vi "main_v1.1.vi"() -> ()   [LabVIEW 2012]
uses:
  SensorSettingCtl.ctl
  SensorTypes.ctl
  states.ctl
  globalVariables.vi
  <vilib>/Analysis/baseanly.llb/Mean (DBL).vi
  <vilib>/Analysis/NI_AALBase.lvlib
panel:
  out "times":dbl[](array[numeric])
  out "diff":dbl
  in  "max. meas. time / ms":dbl=3000.0
  out "means":dbl[](array[numeric])
  out "measuring":bool
  out "i_e":i32
  out "i_s":i32
  out "XY Graph raw":cluster{dbl[], dbl[]}[](graph)
  out "XY Graph":cluster{dbl[], dbl[]}[](graph)
  in  "size of buffer":i32=1000000
  in  "Path for measuring results":path=path "C:/Users/Induelec/Desktop/test_output"
  in  "Sensor types":T1[](array[typedef])=[enum."ITL 900 (Analogue)", enum."CAB 300-C SP3 (CAN)", enum."xyz TODO (PWM)", enum."xyz TODO (LIN)", enum."xyz TODO (Analogue)"]
  in  "Array 2":T2[](array[typedef])=[{"VISA resource name"="", "use sensor"=FALSE}, {"VISA resource name"="", "use sensor"=TRUE}, {"VISA resource name"="", "use sensor"=FALSE}, {"VISA resource name"="", "use sensor"=FALSE}, {"VISA resource name"="", "use sensor"=FALSE}]
  in  "cancel button":bool
  in  "start Button":bool
  out "Error Flag":bool
  # "Measurement of Current Sensors from LEM"
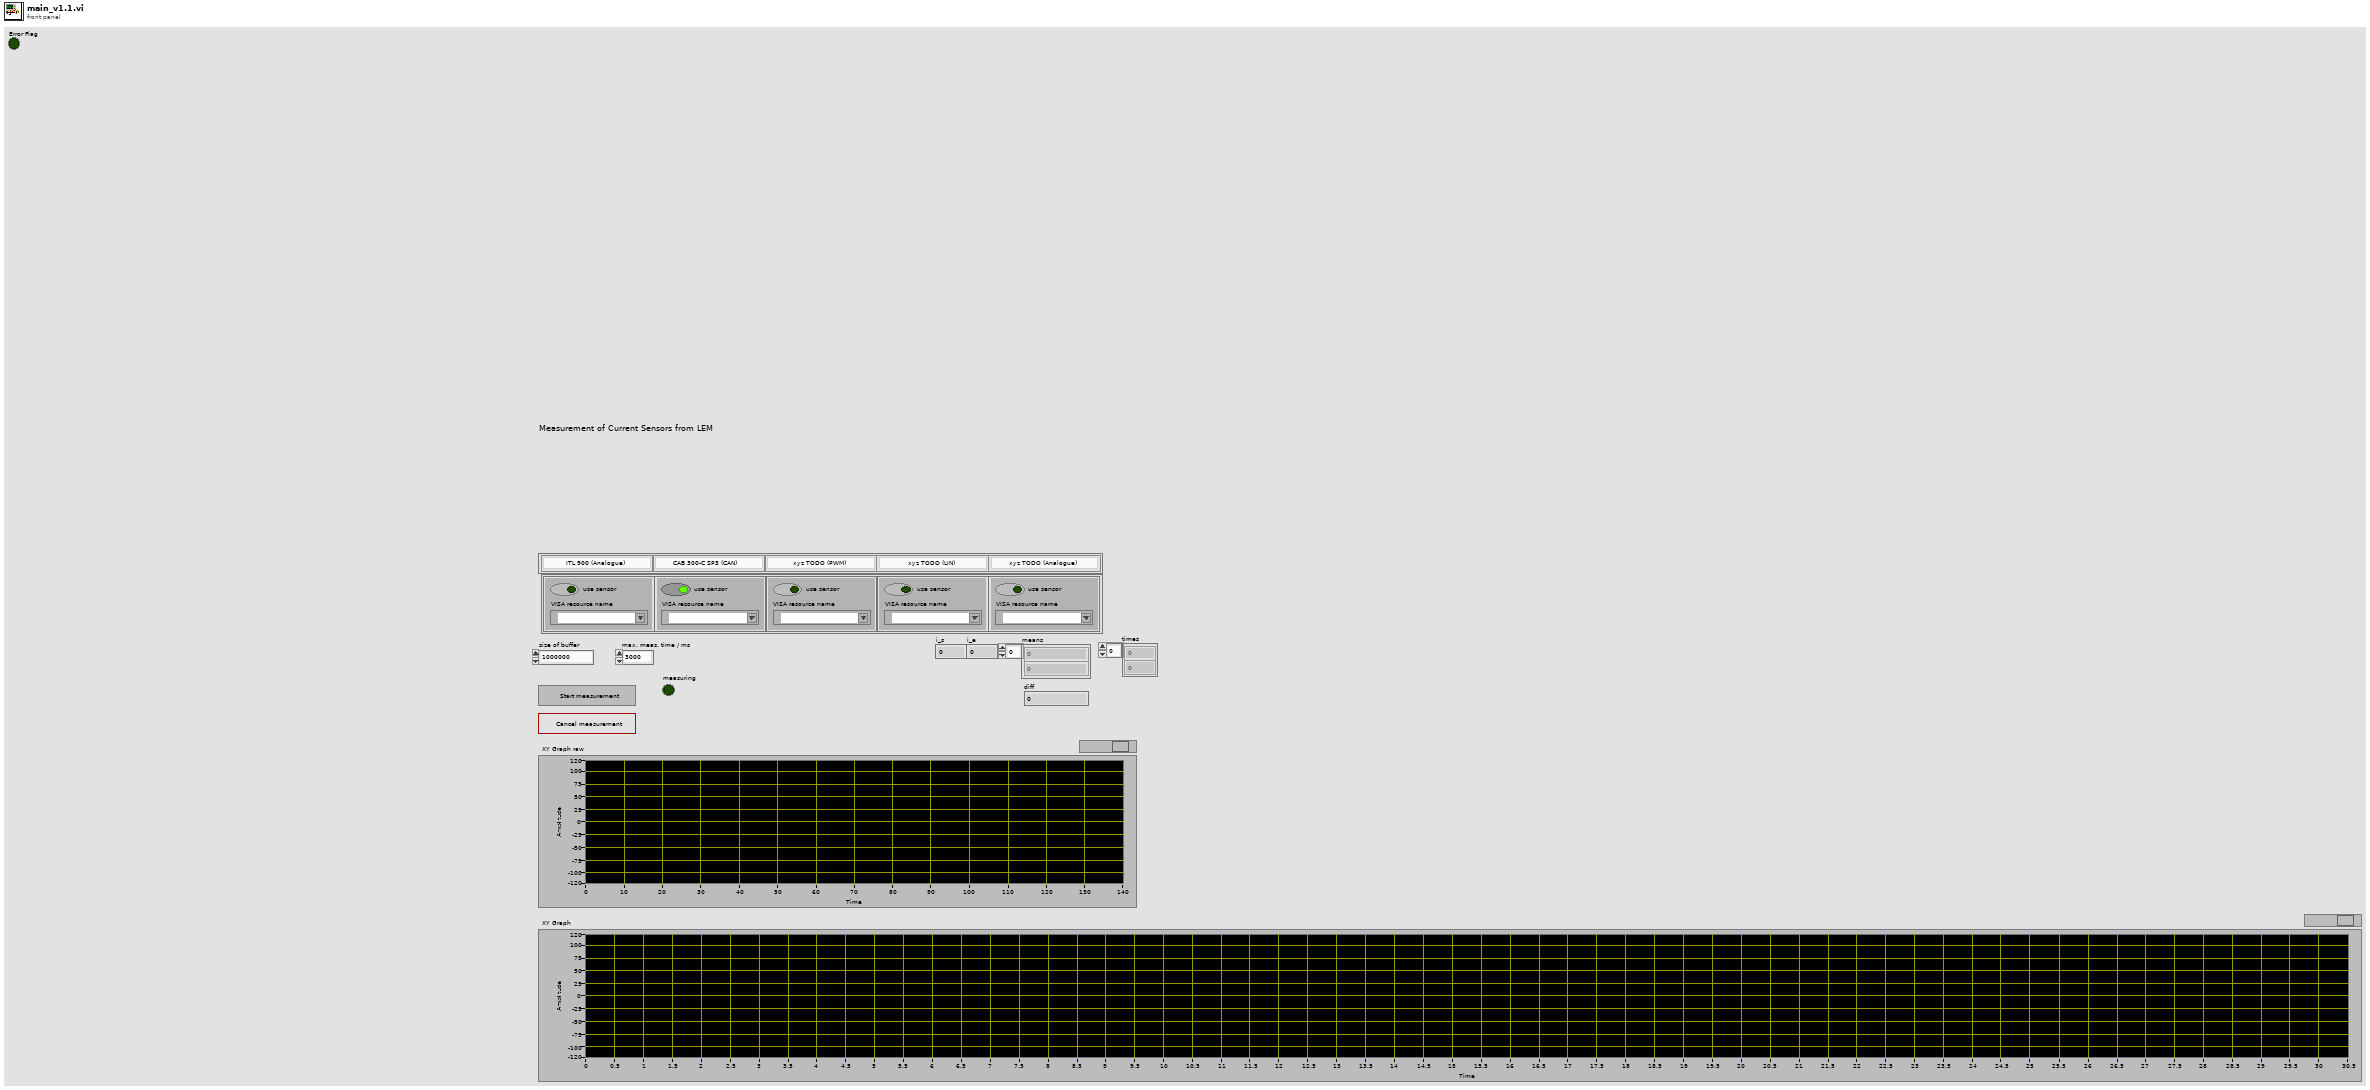
[diagram p1: front panel]
types:
  T1 = typedef "SensorTypes.ctl" = enum16{"ITL 900 (Analogue)", "CAB 300-C SP3 (CAN)", "xyz TODO (PWM)", "xyz TODO (LIN)", "xyz TODO (Analogue)"}
  T2 = typedef "SensorSettingCtl.ctl" = cluster{"VISA resource name":refnum<visa-resource-name>, "use sensor":bool}
  T3 = typedef "states.ctl" = enum16{"init", "wait for user confirm", "start sensors", "measure", "data analysis", "terminate"}
  T4 = typedef "TimeValue.ctl" = cluster{"Time of measurement":timestamp, "Current value":dbl}
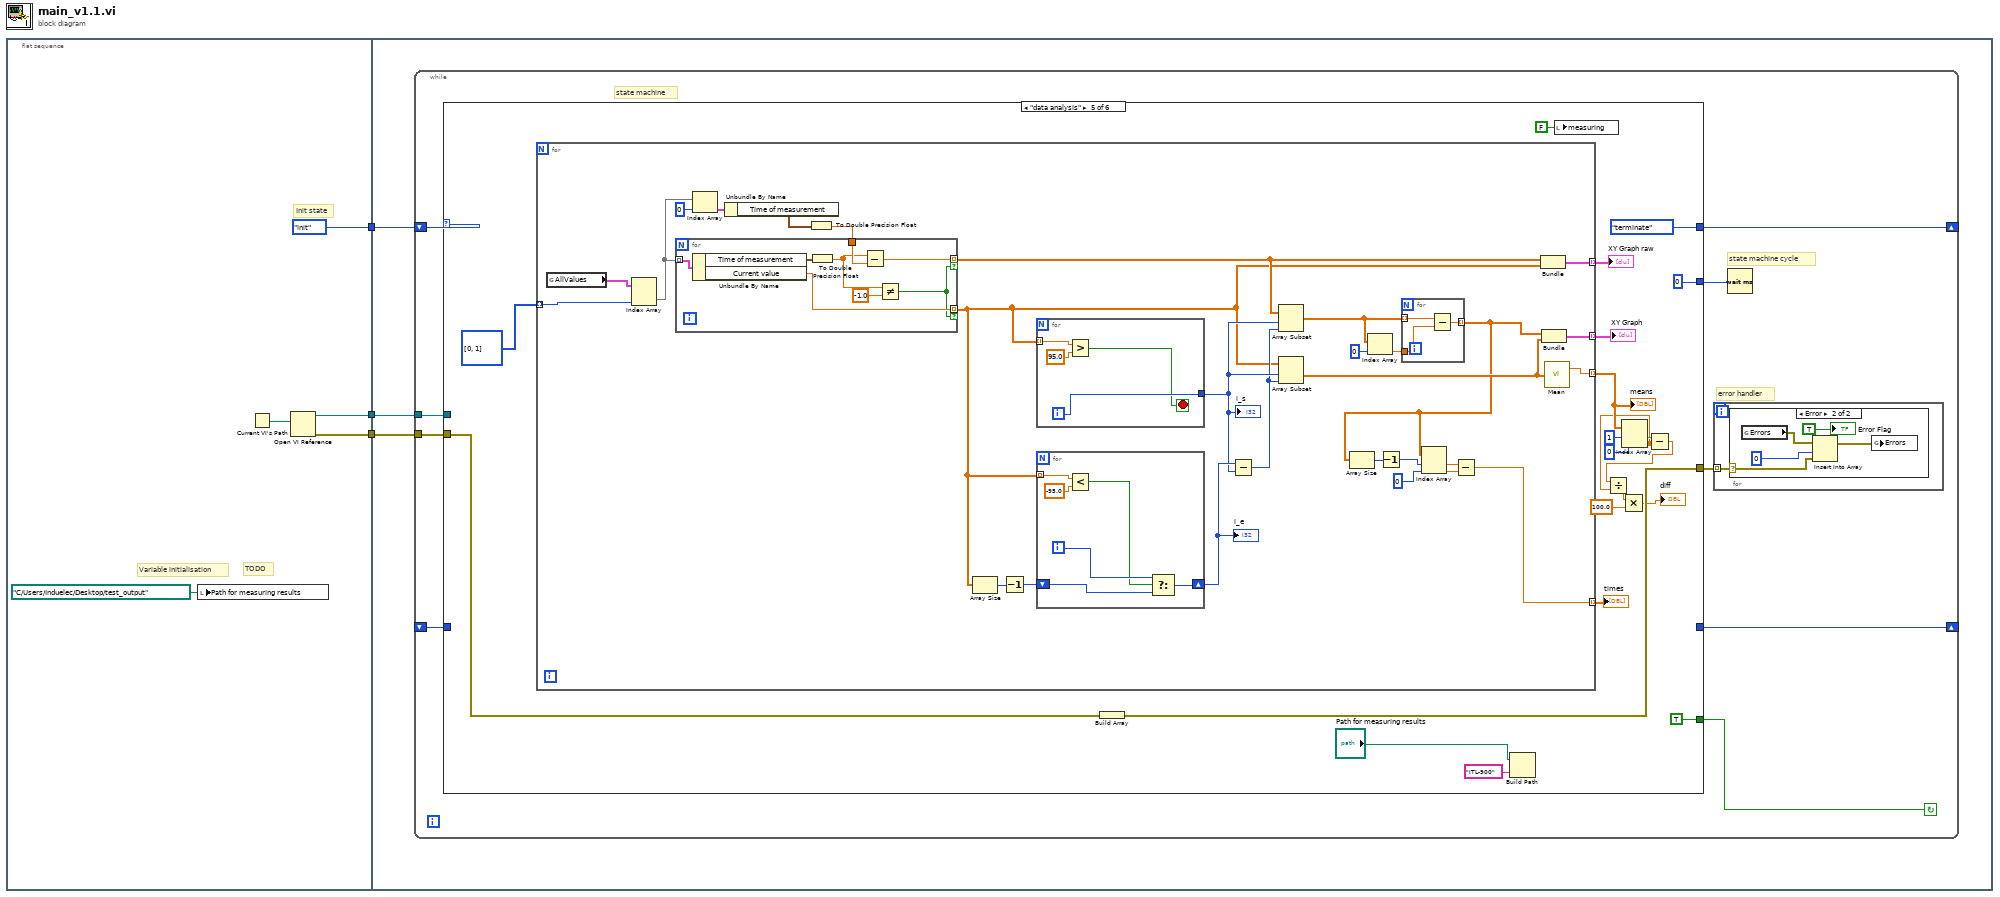
[diagram p0: block diagram]
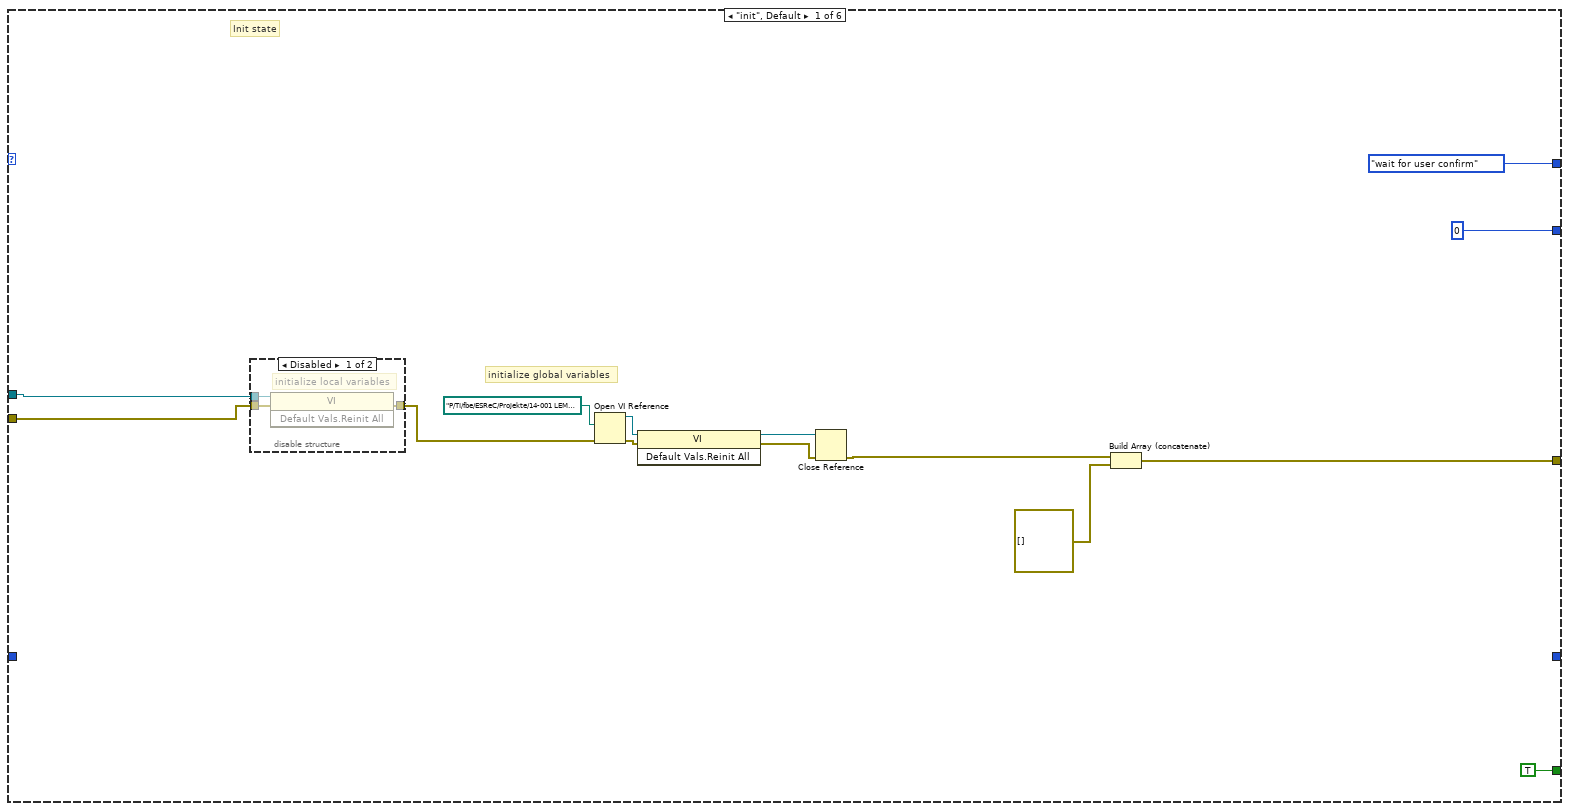
[diagram p3: hidden frame]
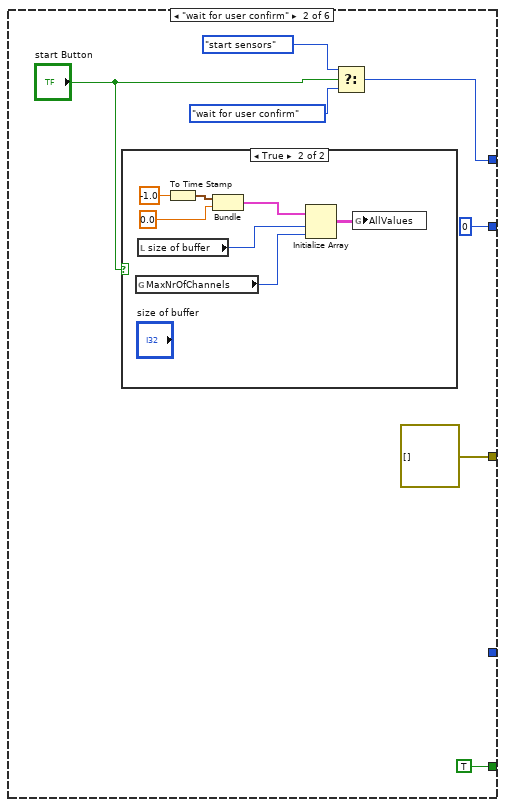
[diagram p5: hidden frame]
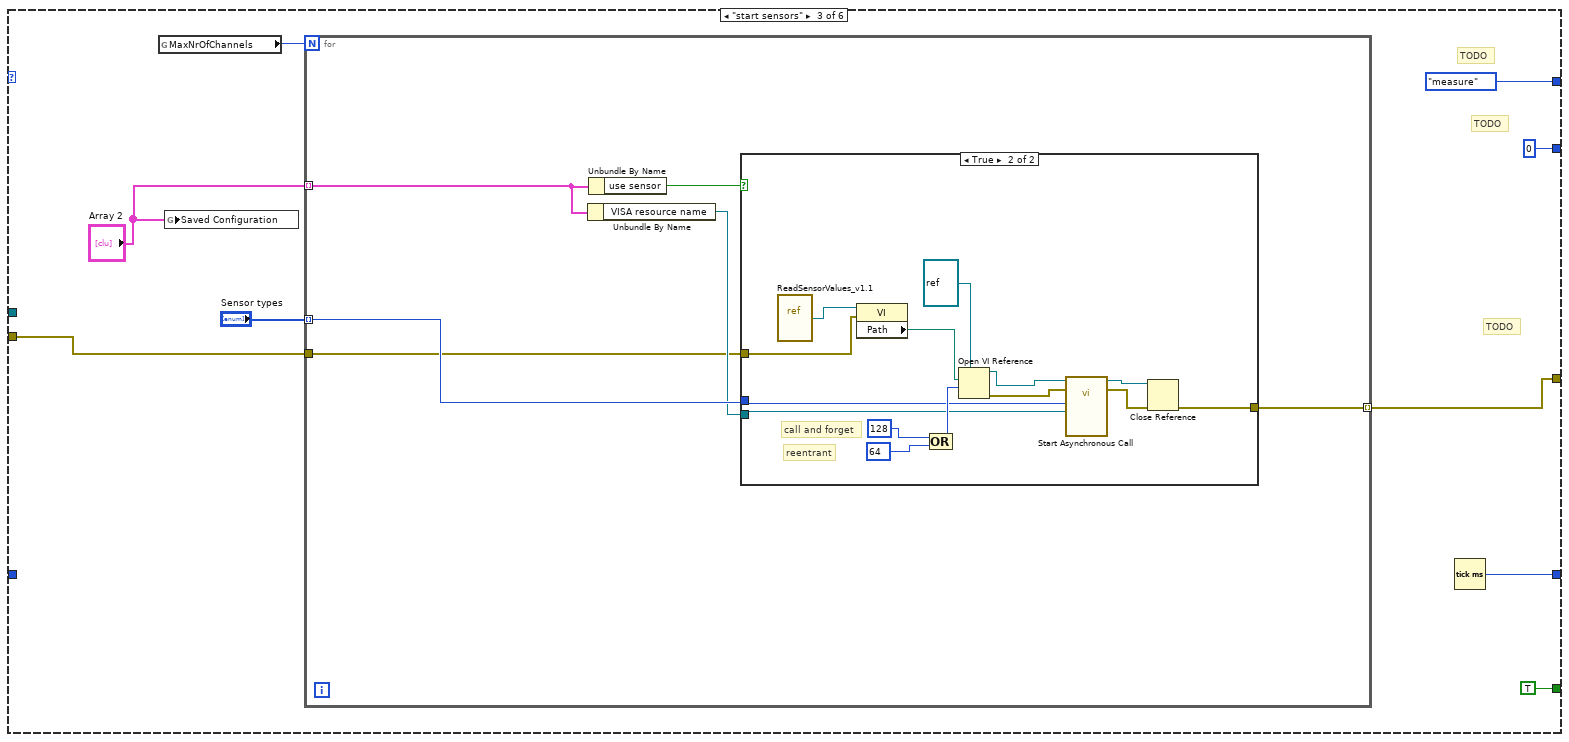
[diagram p7: hidden frame]
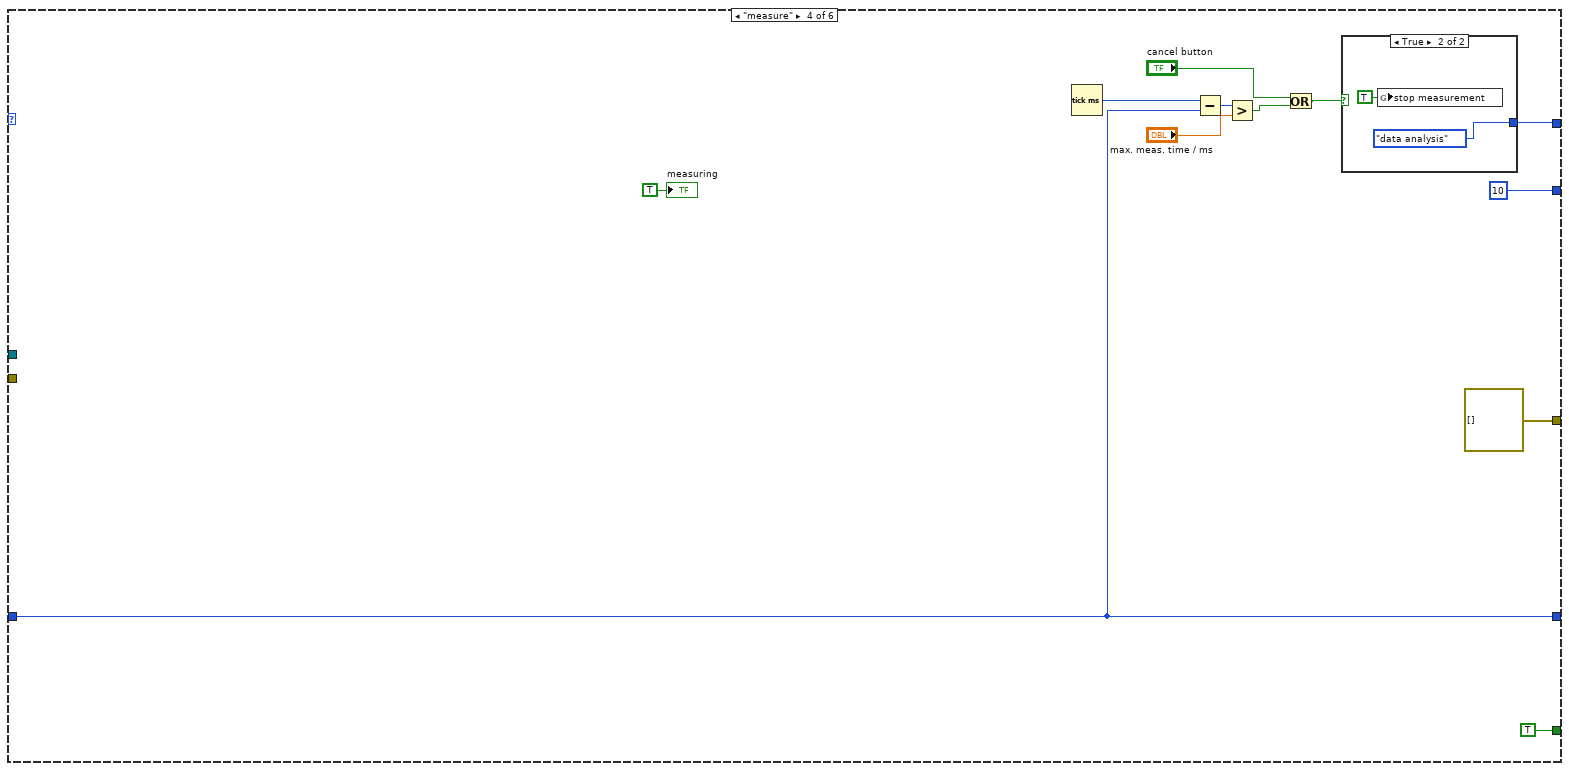
[diagram p9: hidden frame]
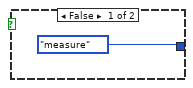
[diagram p10: hidden frame]
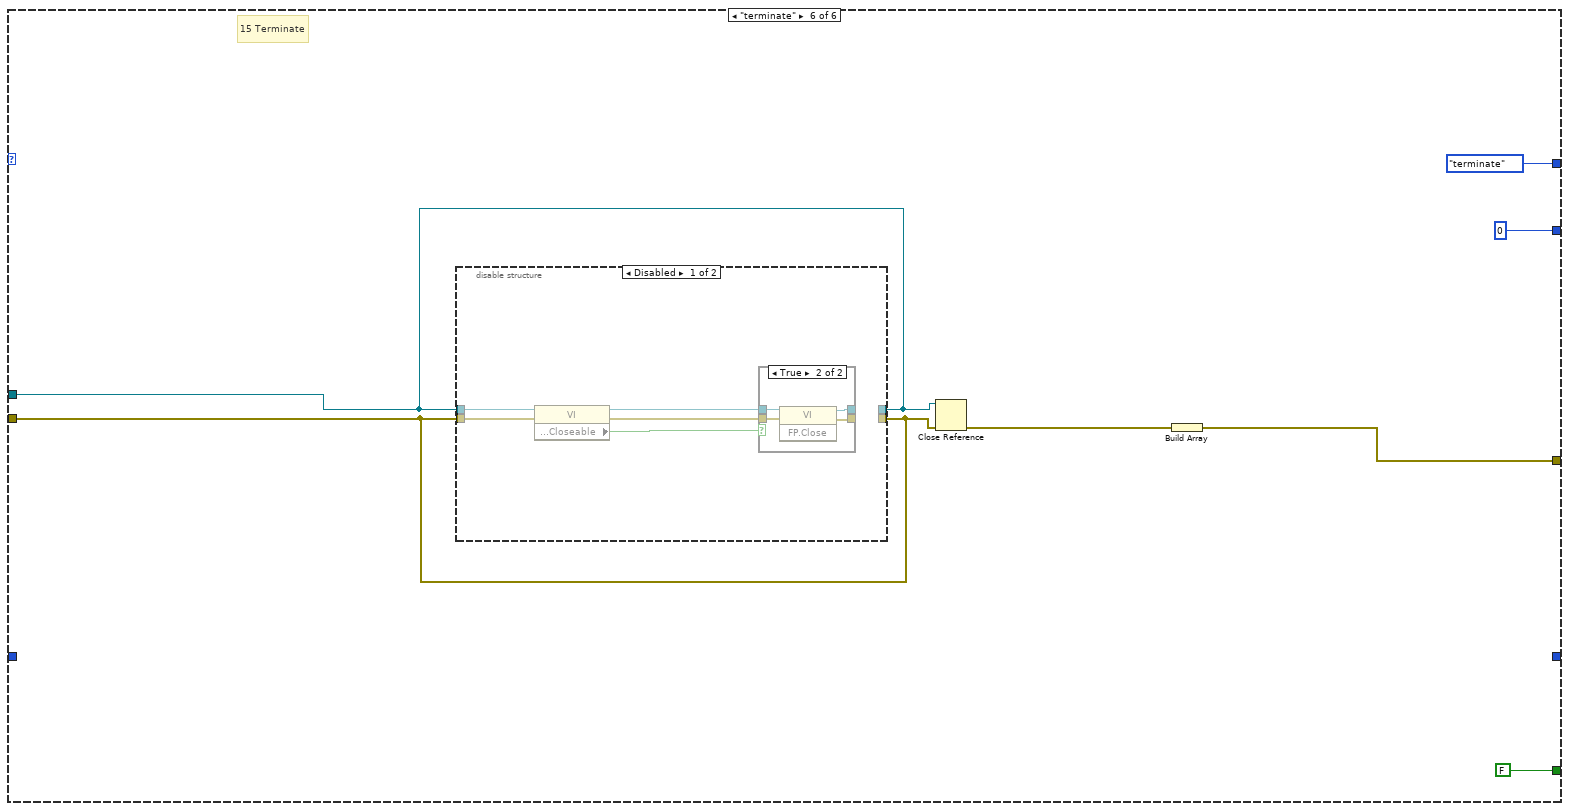
[diagram p11: hidden frame]
diagram:
  n1 = flat-sequence {
    tunnel: [states."init" ("States IEEE-488")] -> w3
    tunnel: [w8] -> w2
    tunnel: [w7] -> w1
    tunnel: w3 -> [w9]
    tunnel: w2 -> [w11]
    tunnel: w1 -> [w10]
    frame #0 {
      # "TODO"
      # "Variable initialisation"
      # "Init state"
      n2 = local write "Path for measuring results"(path "C:/Users/Induelec/Desktop/test_output" ("Path for measuring results")) -> ()
      n3 = Current VI's Path() -> (path=w6:path)
      n4 = Open VI Reference(vi path=w6) -> (vi reference=w8:refnum<vi>, error out=w7:errorcluster)  [unwired: 2 in, 3 out]
    }
    frame #1 {
      n5 = while {
        tunnel: w11 -> [w19]
        tunnel: w10 -> [w18]
        shift-right: [w15] -> _
        shift-left: w9 -> [w16]
        shift-right: [w13] -> _
        shift-left: _ -> [w12]
        stop <- w14 continue-if-true
        # "state machine"
        # "error handler"
        # "state machine cycle"
        n6 = case shown="\"data analysis\"" w16 {
          tunnel: [u32 0 ("milliseconds to wait") u32 0 ("milliseconds to wait") u32 0 ("milliseconds to wait") u32 10 ("milliseconds to wait") u32 0 ("milliseconds to wait") u32 0 ("milliseconds to wait")] -> w20
          tunnel: w19 -> [w37 _ _ _ _ w174]
          tunnel: w18 -> [w38 _ w59 _ w118 w173]
          tunnel: [w39 errorcluster[] [] w64 errorcluster[] [] w119 w178] -> w17
          tunnel: [states."wait for user confirm" ("States IEEE-488") w48 states."measure" ("States IEEE-488") w98 states."terminate" ("f") states."terminate" ("f")] -> w15
          tunnel: [TRUE TRUE TRUE TRUE TRUE FALSE] -> w14
          tunnel: [_ _ w58 w89 _ _] -> w13
          tunnel: w12 -> [_ _ _ w89 _ _]
          frame "init", Default {
            # "initialize global variables"
            # "Init state"
            n7 = disable-structure shown="Disabled" {
              disable-tunnel: w38 -> [w43 _]
              disable-tunnel: w37 -> [w42 _]
              disable-tunnel: [w41 _] -> w31
              frame Disabled {
                # "initialize local variables"
                n8 = invoke class="VI" method="Default Vals.Reinit All"(reference=w42, error in=w43) -> (error out=w41:errorcluster)  [unwired: 1 in, 2 out]
              }
              frame Enabled {
              }
            }
            n9 = Open VI Reference(vi path=path "P:/TI/fbe/ESReC/Projekte/14-001 LEM Current Sensor Measurements/Software/LabVIEW/Current sensor tests/globalVariables.vi", error in (no error)=w31) -> (vi reference=w32:refnum<vi>, error out=w30:errorcluster)  [unwired: 4 in]
            n10 = invoke class="VI" method="Default Vals.Reinit All"(reference=w32, error in=w30) -> (reference out=w29:refnum<vi>, error out=w28:errorcluster)  [unwired: 1 in, 1 out]
            n11 = Close Reference(reference=w29, error in (no error)=w28) -> (error out=w27:errorcluster)
            n12 = Build Array (concatenate)(w27, errorcluster[] [] ("array")) -> (w39:errorcluster[])
          }
          frame "wait for user confirm" {
            n13 = case shown="True" "start Button" {
              frame False {
              }
              frame True {
                n14 = global read "globalVariables.vi" "MaxNrOfChannels"() -> (w57:i32)
                n15 = local read "size of buffer"() -> (w55:i32)
                n16 = To Time Stamp(1:-1.0 ("number")) -> (0:w53:timestamp)
                n17 = Bundle(w53, 0.0) -> (w51:cluster{timestamp, dbl})  [unwired: 1 in]
                n18 = Initialize Array(w51, w55, w57) -> (w56:cluster{timestamp, dbl}[][])
                n19 = global write "globalVariables.vi" "AllValues"(w56) -> ()
              }
            }
            n20 = Select(t=states."start sensors" ("States IEEE-488"), s="start Button", f=states."wait for user confirm" ("States IEEE-488")) -> (s? t:f=w48:T3)
          }
          frame "start sensors" {
            # "TODO"
            # "TODO"
            # "TODO"
            n21 = global read "globalVariables.vi" "MaxNrOfChannels"() -> (w61:i32)
            n22 = global write "globalVariables.vi" "Saved Configuration"("Array 2") -> ()
            n23 = for {
              N: w61 -> [_]
              tunnel: "Array 2" -> [w71] mode=indexing
              tunnel: [w70] -> w64 mode=indexing
              tunnel: "Sensor types" -> [w69] mode=indexing
              tunnel: w59 -> [w67]
              n24 = Unbundle By Name(w71) -> ("VISA resource name"=w68:refnum<visa-resource-name>)
              n25 = Unbundle By Name(w71) -> ("use sensor"=w72:bool)
              n26 = case shown="True" w72 {
                tunnel: [w73 w85] -> w70
                tunnel: w69 -> [_ w76]
                tunnel: w68 -> [_ w75]
                tunnel: w67 -> [w73 w77]
                frame False {
                }
                frame True {
                  # "reentrant"
                  # "call and forget"
                  n27 = vi-ref "ReadSensorValues_v1.1.vi"() -> (w78:refnum<vi>)
                  n28 = property class="VI"(reference=w78, error in=w77) -> ("Path"=w87:path)  [unwired: 2 out]
                  n29 = Compound Arithmetic op=OR(128 ("options"), 64 ("value")) -> (w84:i32)
                  n30 = Open VI Reference(type specifier VI Refnum (for type only)=refnum<vi> refnum, vi path=w87, options=w84) -> (vi reference=w82:refnum<vi>, error out=w81:errorcluster)  [unwired: 3 in]
                  n31 = call-by-ref "Start Asynchronous Call"(reference=w82, error in=w81, "VISA resource name"=w75, "Sensor type"=w76) -> (reference out=w80:refnum<vi>, error out=w79:errorcluster)  [unwired: 10 in]
                  n32 = Close Reference(reference=w80, error in (no error)=w79) -> (error out=w85:errorcluster)
                }
              }
            }
            n33 = Tick Count (ms)() -> (millisecond timer value=w58:u32)
          }
          frame "measure" {
            n34 = Tick Count (ms)() -> (millisecond timer value=w90:u32)
            n35 = Subtract(x=w90, y=w89) -> (x-y=w92:u32)
            n36 = Greater?(x=w92, y="max. meas. time / ms") -> (0:w93:bool)
            n37 = Or(x="cancel button", y=w93) -> (x .or. y?=w95:bool)
            n38 = case shown="True" w95 {
              tunnel: [states."measure" ("f") states."data analysis" ("States IEEE-488")] -> w98
              frame False {
              }
              frame True {
                n39 = global write "globalVariables.vi" "stop measurement"(TRUE ("stop measurement")) -> ()
              }
            }
            "measuring" <- TRUE ("measuring")
          }
          frame "data analysis" {
            n40 = for {
              tunnel: [w145] -> w114 mode=indexing
              tunnel: i32[] [0, 1] -> [w144] mode=indexing
              tunnel: [w138] -> w115 mode=indexing
              tunnel: [w133] -> w112 mode=indexing
              tunnel: [w126] -> w103 mode=indexing
              n41 = global read "globalVariables.vi" "AllValues"() -> (w151:T4[][])
              n42 = Index Array(array=w151, index (col)=w144) -> (element=w149:T4[])  [unwired: 1 in]
              n43 = Index Array(array=w149, index=0) -> (element=w148:T4)
              n44 = Unbundle By Name(w148) -> ("Time of measurement"=w147:timestamp)
              n45 = To Double Precision Float(number=w147) -> (double precision float=w146:dbl)
              n46 = for {
                tunnel: w149 -> [w172] mode=indexing
                tunnel: [w165] -> w137 mode=indexing if=w166
                tunnel: [w170] -> w132 mode=indexing if=w166
                tunnel: w146 -> [w169]
                n47 = Unbundle By Name(w172) -> ("Time of measurement"=w171:timestamp, "Current value"=w170:dbl)
                n48 = To Double Precision Float(number=w171) -> (double precision float=w167:dbl)
                n49 = Subtract(x=w167, y=w169) -> (x-y=w165:dbl)
                n50 = Not Equal?(x=w167, y=-1.0) -> (x != y?=w166:bool)
              }
              n51 = Array Size(array=w132) -> (size(s)=w143:i32)
              n52 = Decrement(x=w143) -> (x-1=w142:i32)
              n53 = for {
                tunnel: w132 -> [w164] mode=indexing
                tunnel: [w162] -> w140
                i -> [w162]
                stop <- w161 stop-if-true
                n54 = Greater?(x=w164, y=95.0) -> (0:w161:bool)
              }
              "i_s" <- w140
              n55 = for {
                tunnel: w132 -> [w160] mode=indexing
                shift-right: [w158] -> w141
                shift-left: w142 -> [w156]
                i -> [w157]
                n56 = Less?(x=w160, y=-95.0) -> (x < y?=w155:bool)
                n57 = Select(t=w157, s=w155, f=w156) -> (s? t:f=w158:i32)
              }
              "i_e" <- w141
              n58 = Subtract(x=w141, y=w140) -> (x-y=w139:i32)
              n59 = Array Subset(array=w137, index=w140, length=w139) -> (w136:dbl[])
              n60 = Array Subset(array=w132, index=w140, length=w139) -> (w131:dbl[])
              n61 = Index Array(array=w136, index=0) -> (element=w134:dbl)
              n62 = for {
                tunnel: w136 -> [w154] mode=indexing
                tunnel: w134 -> [w153]
                tunnel: [w152] -> w129 mode=indexing
                n63 = Subtract(x=w154, y=w153) -> (x-y=w152:dbl)
              }
              n64 = Array Size(array=w129) -> (size(s)=w125:i32)
              n65 = Decrement(x=w125) -> (x-1=w124:i32)
              n66 = Index Array(array=w129, index #1=w124, index #2=0 ("index")) -> (element #1=w127:dbl, element #2=w130:dbl)
              n67 = Subtract(x=w127, y=w130) -> (x-y=w126:dbl)
              n68 = Bundle(w137, w132) -> (w138:cluster{dbl[], dbl[]})  [unwired: 1 in]
              n69 = Bundle(w129, w131) -> (w145:cluster{dbl[], dbl[]})  [unwired: 1 in]
              n70 = call-poly <vilib>:"Mean.vi"("X"=w131) -> ("mean"=w133:dbl)  [unwired: 1 out]
            }
            "XY Graph" <- w114
            "XY Graph raw" <- w115
            "means" <- w112
            "times" <- w103
            n71 = Build Array(w118) -> (w119:errorcluster[])
            n72 = Build Path(base path="Path for measuring results", name or relative path="ITL-900") -> ()  [unwired: 1 out]
            n73 = local write "measuring"(FALSE ("measuring")) -> ()
            n74 = Index Array(array=w112, index #1=1 ("index"), index #2=0 ("index")) -> (element #1=w109:dbl, element #2=w107:dbl)
            n75 = Subtract(x=w109, y=w107) -> (x-y=w108:dbl)
            n76 = Divide(x=w108, y=w107) -> (x/y=w106:dbl)
            n77 = Multiply(x=w106, y=100.0) -> (x*y=→"diff":dbl)
          }
          frame "terminate" {
            # "15 Terminate"
            n78 = disable-structure shown="Disabled" {
              disable-tunnel: w173 -> [w181 _]
              disable-tunnel: w174 -> [w180 _]
              disable-tunnel: w174 -> [_ _]
              disable-tunnel: w173 -> [_ _]
              frame Disabled {
                n79 = property class="VI"(reference=w180, error in=w181) -> (reference out=w183:refnum<vi>, error out=w182:errorcluster, "Front Panel.Closeable"=w184:bool)
                n80 = case shown="True" w184 {
                  tunnel: w183 -> [w186 w190]
                  tunnel: [w186 w189] -> _
                  tunnel: w182 -> [w185 w188]
                  tunnel: [w185 w187] -> _
                  frame False {
                  }
                  frame True {
                    n81 = invoke class="VI" method="FP.Close"(reference=w190, error in=w188) -> (reference out=w189:refnum<vi>, error out=w187:errorcluster)  [unwired: 1 in, 1 out]
                  }
                }
              }
              frame Enabled {
              }
            }
            n82 = Close Reference(reference=w174, error in (no error)=w173) -> (error out=w176:errorcluster)
            n83 = Build Array(w176) -> (w178:errorcluster[])
          }
        }
        n84 = for {
          tunnel: w17 -> [w21] mode=indexing
          n85 = case shown="Error" w21 {
            selector: w21 -> [_ w25]
            frame No Error {
            }
            frame Error {
              n86 = global read "globalVariables.vi" "Errors"() -> (w23:errorcluster[])
              n87 = Insert Into Array(array=w23, index=0, new element=w25) -> (w22:errorcluster[])
              n88 = global write "globalVariables.vi" "Errors"(w22) -> ()
              "Error Flag" <- TRUE ("Error Flag")
            }
          }
        }
        n89 = Wait (ms)(milliseconds to wait=w20) -> ()  [unwired: 1 out]
      }
    }
  }
